vi "Handle Error.vi"(8 "error in (no error)":errorcluster, 11 "Arduino_Stepper in":refnum<class "Arduino_Stepper.lvclass">) -> (0 "error out":errorcluster, 2 "stop actor?":bool=TRUE, 3 "Arduino_Stepper out":refnum<class "Arduino_Stepper.lvclass">)   [LabVIEW 2023, in "Arduino_TranslationStage_UI.lvlib" / "Arduino_Stepper.lvclass"]
doc: "(<B>Filename</B>: Actor Framework.lvlib:Actor.lvclass:Handle Error.vi)\n\nDefines how the actor handles an error that occurred while processing a message. By default, this method does nothing except stop the actor."
uses:
  Arduino_Stepper.lvclass
  Arduino_Stepper.lvclass/Arduino_Stepper.ctl
  <vilib>/ActorFramework/Actor/Actor.lvclass
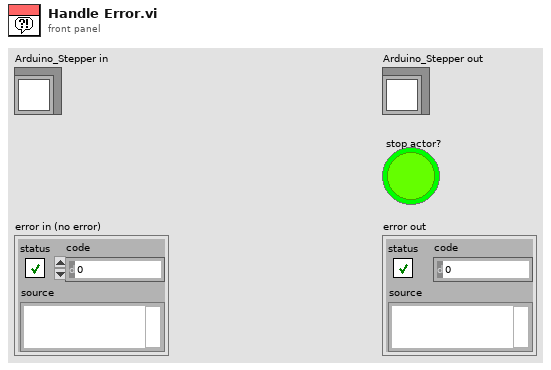
[diagram p1: front panel]
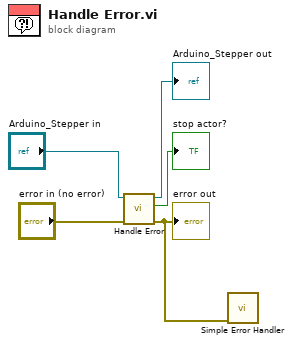
[diagram p0: block diagram]
diagram:
  n1 = call-parent "Handle Error.vi"("error in (no error)"="error in (no error)", "Actor in"="Arduino_Stepper in") -> ("error out"=w1:errorcluster, "stop actor?"=→"stop actor?":bool, "Actor out"=→"Arduino_Stepper out":refnum<class "Arduino_Stepper.lvclass">)  [unwired: 7 in]
  "error out" <- w1
  n2 = call <vilib>:"Simple Error Handler.vi"("error in (no error)"=w1) -> ()  [unwired: 4 in, 5 out]
